vi "StartAsGRPC.vi"(8 "error in":errorcluster, 11 "Service Details":T1) -> (0 "error out":errorcluster, 3 "MicronClient out":refnum<class "MicronClient.lvclass">)   [LabVIEW 2019, in "MicronGRPCClient.lvclass"]
uses:
  MicronGRPCClient.lvclass
  Base/Client/MicronClient.lvclass
  D:/GitHub/KarthikAbiram/Micron/LabVIEW/Source/vi.lib/Micron/Base/Client/MicronClient.lvclass
  Base/Client/Typedefs/ServiceDetails.ctl
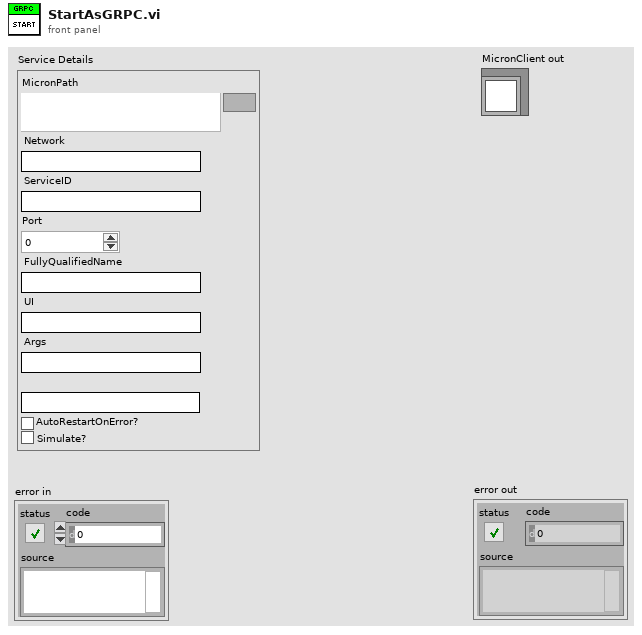
[diagram p1: front panel]
types:
  T1 = typedef "MicronClient.lvclass/ServiceDetails.ctl" = cluster{"MicronPath":path, "Network":string, "ServiceID":string, "Port":i32, "FullyQualifiedName":string, "UI":string, "Args":string, "Mode":string, "AutoRestartOnError?":bool, "Simulate?":bool}
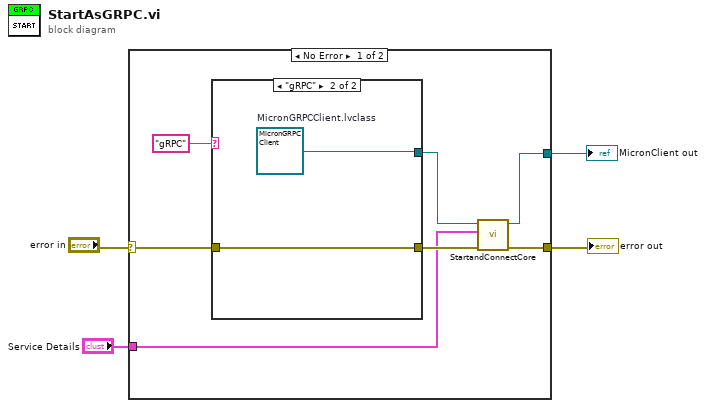
[diagram p0: block diagram]
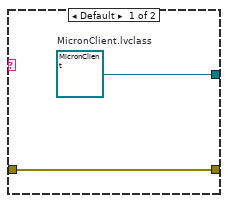
[diagram p2: hidden frame]
diagram:
  n1 = case shown="No Error" "error in" {
    selector: "error in" -> [w7 w16]
    tunnel: [w10 w16] -> w3
    tunnel: [w9 _] -> w2
    tunnel: "Service Details" -> [w5 _]
    frame No Error {
      n2 = case shown="\"gRPC\"" "gRPC" {
        tunnel: [w13 w15] -> w8
        tunnel: w7 -> [w12 w14]
        tunnel: [w12 w14] -> w6
        frame Default {
          w13 = refnum<class "MicronClient.lvclass"> refnum  # MicronClient.lvclass
        }
        frame "gRPC" {
          w15 = refnum<class "MicronGRPCClient.lvclass"> refnum  # MicronGRPCClient.lvclass
        }
      }
      n3 = call-dynamic "StartandConnectCore.vi"("error in (no error)"=w6, "Service Details"=w5, "MicronClient in"=w8) -> ("error out"=w10:errorcluster, "MicronClient out"=w9:refnum<class "MicronClient.lvclass">)  [unwired: 7 in]
    }
    frame Error {
    }
  }
  "error out" <- w3
  "MicronClient out" <- w2
